vi "Time-str-array-to-time-dbl-array.vi"(1 "Array-str":string[](array[string])) -> (0 "Array-dbl":dbl[](array[numeric]) format="%.6g")   [LabVIEW 2019]
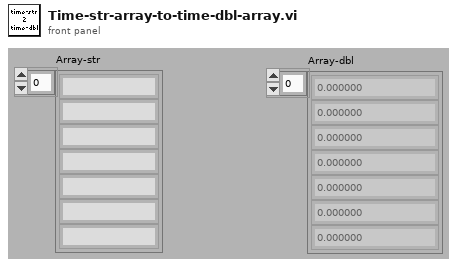
[diagram p1: front panel]
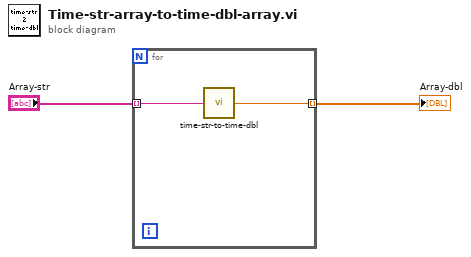
[diagram p0: block diagram]
diagram:
  n1 = for {
    tunnel: "Array-str" -> [w4] mode=indexing
    tunnel: [w3] -> w1 mode=indexing
    n2 = call "time-str-to-time-dbl.vi"("Chaîne"=w4) -> ("TCS_coords"=w3:dbl)
  }
  "Array-dbl" <- w1
